vi "Get Version from Build Spec.vi"() -> (0 "error out":errorcluster, 1 "Version Number":u32, 2 "Version":T1, 3 "Version String":string)   [LabVIEW 2023]
uses:
  <vilib>/AppBuilder/AB_API_Simple/Build Specification Version.ctl
  <vilib>/AppBuilder/AB_API_Simple/NI_App_Builder_API.lvlib
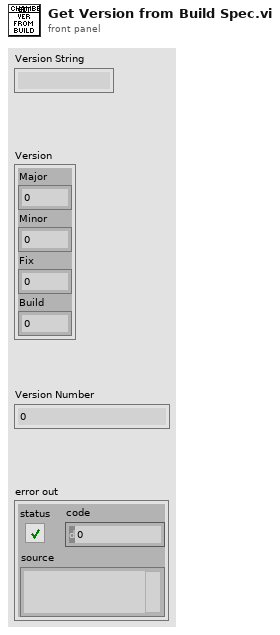
[diagram p1: front panel]
types:
  T1 = typedef "NI_App_Builder_API.lvlib/Build Specification Version.ctl" = cluster{"Major":u16, "Minor":u16, "Fix":u16, "Build":u16}
  T2 = cluster{"Major":u16, "Minor":u16, "Fix":u16, "Build":u16}
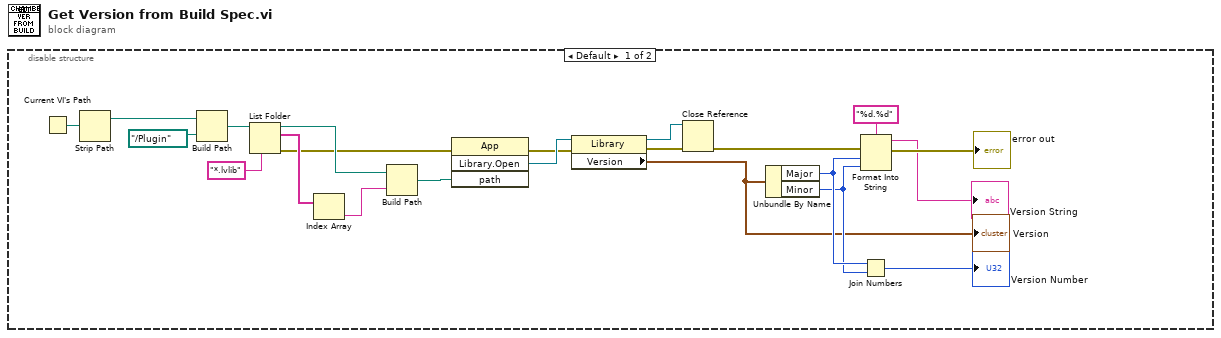
[diagram p0: block diagram]
diagram:
  n1 = disable-structure shown="Default" {
    frame condition #0 (active) {
      n2 = Current VI's Path() -> (path=w22:path)
      n3 = Strip Path(path=w22) -> (stripped path=w18:path)  [unwired: 1 out]
      n4 = Build Path(base path=w18, name or relative path=path "../Plugin") -> (appended path=w20:path)
      n5 = List Folder(path=w20, pattern="*.lvlib") -> (path out=w9:path, filenames=w11:string[], error out=w7:errorcluster)  [unwired: 2 in, 1 out]
      n6 = Index Array(array=w11) -> (element=w10:string)  [unwired: 1 in]
      n7 = Build Path(base path=w9, name or relative path=w10) -> (appended path=w8:path)
      n8 = invoke class="App" method="Library.Open"(error in=w7, "path"=w8) -> (error out=w5:errorcluster, "Open Library"=w6:refnum<vi>)  [unwired: 2 in, 2 out]
      n9 = property class="Library"(reference=w6, error in=w5) -> (reference out=w2:refnum<vi>, error out=w4:errorcluster, "Version"=w1:T2)
      "Version" <- w1
      n10 = Close Reference(reference=w2, error in (no error)=w4) -> (error out=w3:errorcluster)
      n11 = Unbundle By Name(w1) -> ("Major"=w14:u16, "Minor"=w13:u16)
      n12 = Format Into String(format string="%d.%d", error in=w3, w14, w13) -> (resulting string=→"Version String":string, error out=→"error out":errorcluster)  [unwired: 1 in]
      n13 = Join Numbers(hi=w14, lo=w13) -> ((hi.lo)=→"Version Number":u32)
    }
    frame condition #1 {
    }
  }
